vi "Lift Init.vi"   [LabVIEW 2014]
uses:
  Begin/Global Variables.vi
  Begin/Global RefNums.vi
types:
  T1 = typedef "WPI_SwitchDevRef.ctl" = cluster{"DevStatus":errorcluster, "DIO Channel":T2, "Controller":T3, "CntIndex":T4, "Normally Closed":bool}
  T2 = typedef "FPGA_DIOChannel.ctl" = enum8{"DIO 0", "DIO 1", "DIO 2", "DIO 3", "DIO 4", "DIO 5", "DIO 6", "DIO 7", "DIO 8", "DIO 9", "DIO MXP 0", "DIO MXP 1", "DIO MXP 2", "DIO MXP 3", "DIO MXP 4", "DIO MXP 5", "DIO MXP 6", "DIO MXP 7", "DIO MXP 8", "DIO MXP 9", "DIO MXP 10", "DIO MXP 11", "DIO MXP 12", "DIO MXP 13", "DIO MXP 14", "DIO MXP 15", "Invalid"}
  T3 = typedef "FPGA_TypedefDigitalModule.ctl" = enum16{"Controller 1"}
  T4 = typedef "FPGA_CounterCtrSystemIndex.ctl" = enum8{"Ctr 0", "Ctr 1", "Ctr 2", "Ctr 3", "Ctr 4", "Ctr 5", "Ctr 6", "Ctr 7", "Invalid"}
  T5 = typedef "WPI_MotorControlDeviceRef.ctl" = cluster{"DeviceStatus":errorcluster, "Type":T6, "PWM":cluster{"Controller":T3, "PWM Channel":T7, "DeadBand":T8}, "CAN":cluster{"Device Number":u8, "Control Mode":T9, "Semaphore":T10, "Max Vout":dbl, "TalonSRX Control Mode":T11}, "Invert":bool, "TransformRef":T12, "InvTransformRef":T12}
  T6 = typedef "WPI_MotorControlType.ctl" = enum16{"PWM", "CAN", "CANTalonSRX"}
  T7 = typedef "FPGA_DIOPWMChannel.ctl" = enum8{"PWM 0", "PWM 1", "PWM 2", "PWM 3", "PWM 4", "PWM 5", "PWM 6", "PWM 7", "PWM 8", "PWM 9", "PWM MXP 0", "PWM MXP 1", "PWM MXP 2", "PWM MXP 3", "PWM MXP 4", "PWM MXP 5", "PWM MXP 6", "PWM MXP 7", "PWM MXP 8", "PWM MXP 9", "Invalid"}
  T8 = typedef "WPI_PWMDeadband.ctl" = cluster{"Name":string, "maxPositivePwm":i32, "minPositivePwm":i32, "centerPwm":i32, "maxNegativePwm":i32, "minNegativePwm":i32, "angularRange":u16}
  T9 = typedef "WPI_CANJaguar_ControlMode.ctl" = enum8{"Percent VBus", "Current", "Speed", "Position", "Voltage"}
  T10 = typedef "Semaphore RefNum" = refnum<k1>
  T11 = typedef "WPI_CANTalonSRX_APIControlMode.ctl" = enum8{"Percent VBus", "Speed", "Position", "Slave", "Unchanged / Invalid"}
  T12 = typedef "WPI_PWMTransform_ConPane.ctl" = refnum<vi>
  T13 = typedef "WPI_EncoderDevRef.ctl" = cluster{"DevStatus":errorcluster, "EncoderIndex":T14, "CounterIndex":T4, "DistancePerCount":dbl, "Decoding Type":T15}
  T14 = typedef "FPGA_EncoderIdx.ctl" = enum8{"Enc 0", "Enc 1", "Enc 2", "Enc 3", "Enc 4", "Enc 5", "Enc 6", "Enc 7", "Invalid"}
  T15 = typedef "WPI_EncoderType.ctl" = enum16{"1x", "2x", "4x"}
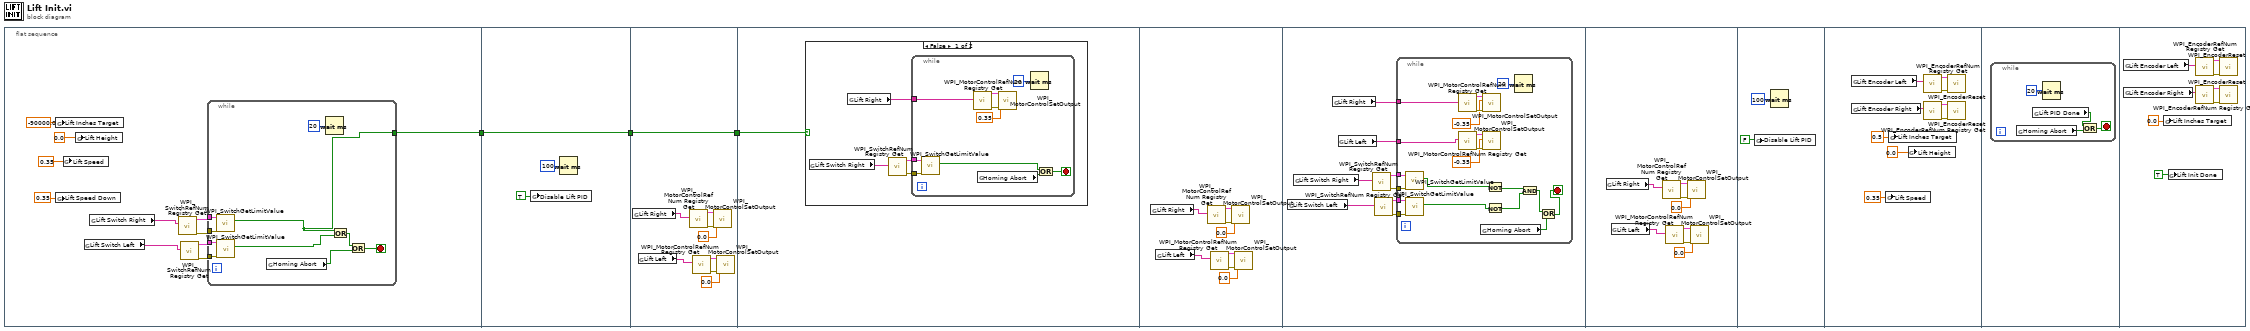
[diagram p0: block diagram]
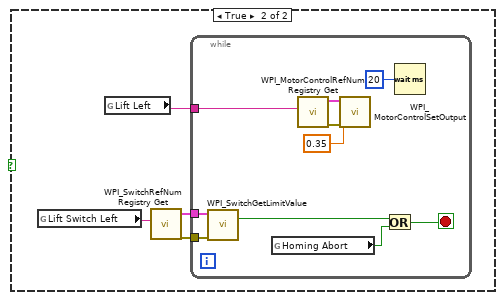
[diagram p2: hidden frame]
diagram:
  n1 = flat-sequence {
    tunnel: [w5] -> w2
    tunnel: w2 -> [w27]
    tunnel: [w27] -> w1
    tunnel: w1 -> [w36]
    tunnel: [w36] -> w3
    tunnel: w3 -> [w37]
    frame #0 {
      n2 = global write "Global Variables.vi" "Lift Inches Target"(-90000.0 ("Lift Inches Target")) -> ()
      n3 = global write "Global Variables.vi" "Lift Speed Down"(0.35 ("Lift Speed Down")) -> ()
      n4 = global write "Global Variables.vi" "Lift Speed"(0.35 ("t")) -> ()
      n5 = global write "Global Variables.vi" "Lift Height"(0.0 ("Lift Inches Target")) -> ()
      n6 = global read "Global RefNums.vi" "Lift Switch Left"() -> (w10:string)
      n7 = global read "Global RefNums.vi" "Lift Switch Right"() -> (w11:string)
      n8 = call <vilib>:"WPI_SwitchRefNum Registry Get.vi"("refnum name"=w11) -> ("error out"=w8:errorcluster, "SwitchDevRef"=w9:T1)  [unwired: 9 in]
      n9 = call <vilib>:"WPI_SwitchRefNum Registry Get.vi"("refnum name"=w10) -> ("error out"=w7:errorcluster, "SwitchDevRef"=w6:T1)  [unwired: 9 in]
      n10 = while {
        tunnel: w9 -> [w23]
        tunnel: w8 -> [w22]
        tunnel: w6 -> [w21]
        tunnel: w7 -> [w20]
        tunnel: [w18] -> w5
        stop <- w15 stop-if-true
        n11 = call <vilib>:"WPI_SwitchGetLimitValue.vi"("error in (no error)"=w22, "SwitchDevRef"=w23) -> ("Switch Pressed"=w18:bool)  [unwired: 7 in, 2 out]
        n12 = call <vilib>:"WPI_SwitchGetLimitValue.vi"("error in (no error)"=w20, "SwitchDevRef"=w21) -> ("Switch Pressed"=w19:bool)  [unwired: 7 in, 2 out]
        n13 = global read "Global Variables.vi" "Homing Abort"() -> (w17:bool)
        n14 = Wait (ms)(milliseconds to wait=u32 20) -> ()  [unwired: 1 out]
        n15 = Or(x=w18, y=w19) -> (x .or. y?=w16:bool)
        n16 = Or(x=w16, y=w17) -> (x .or. y?=w15:bool)
      }
    }
    frame #1 {
      n17 = global write "Global Variables.vi" "Disable Lift PID"(TRUE ("Disable Lift PID")) -> ()
      n18 = Wait (ms)(milliseconds to wait=u32 100) -> ()  [unwired: 1 out]
    }
    frame #2 {
      n19 = global read "Global RefNums.vi" "Lift Right"() -> (w33:string)
      n20 = global read "Global RefNums.vi" "Lift Left"() -> (w29:string)
      n21 = call <vilib>:"WPI_MotorControlRefNum Registry Get.vi"("refnum name"=w33) -> ("error out"=w35:errorcluster, "MotorControlDevRef"=w32:T5)  [unwired: 9 in]
      n22 = call <vilib>:"WPI_MotorControlRefNum Registry Get.vi"("refnum name"=w29) -> ("error out"=w31:errorcluster, "MotorControlDevRef"=w28:T5)  [unwired: 9 in]
      n23 = call <vilib>:"WPI_MotorControlSetOutput.vi"("error in (no error)"=w35, "Output"=0.0, "MotorControlDevRef"=w32) -> ()  [unwired: 6 in, 3 out]
      n24 = call <vilib>:"WPI_MotorControlSetOutput.vi"("error in (no error)"=w31, "Output"=0.0, "MotorControlDevRef"=w28) -> ()  [unwired: 6 in, 3 out]
    }
    frame #3 {
      n25 = case shown="False" w37 {
        frame False {
          n26 = global read "Global RefNums.vi" "Lift Switch Right"() -> (w40:string)
          n27 = global read "Global RefNums.vi" "Lift Right"() -> (w41:string)
          n28 = call <vilib>:"WPI_SwitchRefNum Registry Get.vi"("refnum name"=w40) -> ("error out"=w38:errorcluster, "SwitchDevRef"=w39:T1)  [unwired: 9 in]
          n29 = while {
            tunnel: w41 -> [w48]
            tunnel: w39 -> [w47]
            tunnel: w38 -> [w46]
            stop <- w42 stop-if-true
            n30 = call <vilib>:"WPI_SwitchGetLimitValue.vi"("error in (no error)"=w46, "SwitchDevRef"=w47) -> ("Switch Pressed"=w43:bool)  [unwired: 7 in, 2 out]
            n31 = call <vilib>:"WPI_MotorControlRefNum Registry Get.vi"("refnum name"=w48) -> ("error out"=w50:errorcluster, "MotorControlDevRef"=w51:T5)  [unwired: 9 in]
            n32 = global read "Global Variables.vi" "Homing Abort"() -> (w44:bool)
            n33 = call <vilib>:"WPI_MotorControlSetOutput.vi"("error in (no error)"=w50, "Output"=0.35, "MotorControlDevRef"=w51) -> ()  [unwired: 6 in, 3 out]
            n34 = Wait (ms)(milliseconds to wait=u32 20) -> ()  [unwired: 1 out]
            n35 = Or(x=w43, y=w44) -> (x .or. y?=w42:bool)
          }
        }
        frame True {
          n36 = global read "Global RefNums.vi" "Lift Switch Left"() -> (w53:string)
          n37 = global read "Global RefNums.vi" "Lift Left"() -> (w52:string)
          n38 = call <vilib>:"WPI_SwitchRefNum Registry Get.vi"("refnum name"=w53) -> ("error out"=w54:errorcluster, "SwitchDevRef"=w55:T1)  [unwired: 9 in]
          n39 = while {
            tunnel: w55 -> [w62]
            tunnel: w54 -> [w61]
            tunnel: w52 -> [w60]
            stop <- w58 stop-if-true
            n40 = call <vilib>:"WPI_SwitchGetLimitValue.vi"("error in (no error)"=w61, "SwitchDevRef"=w62) -> ("Switch Pressed"=w57:bool)  [unwired: 7 in, 2 out]
            n41 = global read "Global Variables.vi" "Homing Abort"() -> (w56:bool)
            n42 = call <vilib>:"WPI_MotorControlRefNum Registry Get.vi"("refnum name"=w60) -> ("error out"=w64:errorcluster, "MotorControlDevRef"=w65:T5)  [unwired: 9 in]
            n43 = call <vilib>:"WPI_MotorControlSetOutput.vi"("error in (no error)"=w64, "Output"=0.35, "MotorControlDevRef"=w65) -> ()  [unwired: 6 in, 3 out]
            n44 = Or(x=w57, y=w56) -> (x .or. y?=w58:bool)
            n45 = Wait (ms)(milliseconds to wait=u32 20) -> ()  [unwired: 1 out]
          }
        }
      }
    }
    frame #4 {
      n46 = global read "Global RefNums.vi" "Lift Right"() -> (w71:string)
      n47 = global read "Global RefNums.vi" "Lift Left"() -> (w67:string)
      n48 = call <vilib>:"WPI_MotorControlRefNum Registry Get.vi"("refnum name"=w71) -> ("error out"=w73:errorcluster, "MotorControlDevRef"=w70:T5)  [unwired: 9 in]
      n49 = call <vilib>:"WPI_MotorControlRefNum Registry Get.vi"("refnum name"=w67) -> ("error out"=w69:errorcluster, "MotorControlDevRef"=w66:T5)  [unwired: 9 in]
      n50 = call <vilib>:"WPI_MotorControlSetOutput.vi"("error in (no error)"=w73, "Output"=0.0, "MotorControlDevRef"=w70) -> ()  [unwired: 6 in, 3 out]
      n51 = call <vilib>:"WPI_MotorControlSetOutput.vi"("error in (no error)"=w69, "Output"=0.0, "MotorControlDevRef"=w66) -> ()  [unwired: 6 in, 3 out]
    }
    frame #5 {
      n52 = global read "Global RefNums.vi" "Lift Switch Left"() -> (w74:string)
      n53 = global read "Global RefNums.vi" "Lift Switch Right"() -> (w80:string)
      n54 = global read "Global RefNums.vi" "Lift Right"() -> (w81:string)
      n55 = global read "Global RefNums.vi" "Lift Left"() -> (w77:string)
      n56 = call <vilib>:"WPI_SwitchRefNum Registry Get.vi"("refnum name"=w80) -> ("error out"=w78:errorcluster, "SwitchDevRef"=w79:T1)  [unwired: 9 in]
      n57 = call <vilib>:"WPI_SwitchRefNum Registry Get.vi"("refnum name"=w74) -> ("error out"=w75:errorcluster, "SwitchDevRef"=w76:T1)  [unwired: 9 in]
      n58 = while {
        tunnel: w81 -> [w98]
        tunnel: w79 -> [w97]
        tunnel: w78 -> [w96]
        tunnel: w77 -> [w92]
        tunnel: w76 -> [w91]
        tunnel: w75 -> [w90]
        stop <- w82 stop-if-true
        n59 = call <vilib>:"WPI_SwitchGetLimitValue.vi"("error in (no error)"=w96, "SwitchDevRef"=w97) -> ("Switch Pressed"=w87:bool)  [unwired: 7 in, 2 out]
        n60 = call <vilib>:"WPI_SwitchGetLimitValue.vi"("error in (no error)"=w90, "SwitchDevRef"=w91) -> ("Switch Pressed"=w85:bool)  [unwired: 7 in, 2 out]
        n61 = call <vilib>:"WPI_MotorControlRefNum Registry Get.vi"("refnum name"=w98) -> ("error out"=w100:errorcluster, "MotorControlDevRef"=w101:T5)  [unwired: 9 in]
        n62 = call <vilib>:"WPI_MotorControlRefNum Registry Get.vi"("refnum name"=w92) -> ("error out"=w94:errorcluster, "MotorControlDevRef"=w89:T5)  [unwired: 9 in]
        n63 = global read "Global Variables.vi" "Homing Abort"() -> (w84:bool)
        n64 = call <vilib>:"WPI_MotorControlSetOutput.vi"("error in (no error)"=w100, "Output"=-0.35 ("right side  2"), "MotorControlDevRef"=w101) -> ()  [unwired: 6 in, 3 out]
        n65 = call <vilib>:"WPI_MotorControlSetOutput.vi"("error in (no error)"=w94, "Output"=-0.35 ("right side  2"), "MotorControlDevRef"=w89) -> ()  [unwired: 6 in, 3 out]
        n66 = Not(x=w87) -> (.not. x?=w88:bool)
        n67 = Not(x=w85) -> (.not. x?=w86:bool)
        n68 = Wait (ms)(milliseconds to wait=u32 20) -> ()  [unwired: 1 out]
        n69 = And(x=w88, y=w86) -> (x .and. y?=w83:bool)
        n70 = Or(x=w83, y=w84) -> (x .or. y?=w82:bool)
      }
    }
    frame #6 {
      n71 = global read "Global RefNums.vi" "Lift Right"() -> (w107:string)
      n72 = global read "Global RefNums.vi" "Lift Left"() -> (w103:string)
      n73 = call <vilib>:"WPI_MotorControlRefNum Registry Get.vi"("refnum name"=w107) -> ("error out"=w109:errorcluster, "MotorControlDevRef"=w106:T5)  [unwired: 9 in]
      n74 = call <vilib>:"WPI_MotorControlRefNum Registry Get.vi"("refnum name"=w103) -> ("error out"=w105:errorcluster, "MotorControlDevRef"=w102:T5)  [unwired: 9 in]
      n75 = call <vilib>:"WPI_MotorControlSetOutput.vi"("error in (no error)"=w109, "Output"=0.0, "MotorControlDevRef"=w106) -> ()  [unwired: 6 in, 3 out]
      n76 = call <vilib>:"WPI_MotorControlSetOutput.vi"("error in (no error)"=w105, "Output"=0.0, "MotorControlDevRef"=w102) -> ()  [unwired: 6 in, 3 out]
    }
    frame #7 {
      n77 = global write "Global Variables.vi" "Disable Lift PID"(FALSE ("Disable Lift PID")) -> ()
      n78 = Wait (ms)(milliseconds to wait=u32 100) -> ()  [unwired: 1 out]
    }
    frame #8 {
      n79 = global read "Global RefNums.vi" "Lift Encoder Left"() -> (w117:string)
      n80 = global read "Global RefNums.vi" "Lift Encoder Right"() -> (w116:string)
      n81 = global write "Global Variables.vi" "Lift Speed"(0.35 ("Lift Speed")) -> ()
      n82 = global write "Global Variables.vi" "Lift Inches Target"(0.5 ("Lift Inches Target")) -> ()
      n83 = global write "Global Variables.vi" "Lift Height"(0.0 ("Lift Inches Target")) -> ()
      n84 = call <vilib>:"WPI_EncoderRefNum Registry Get.vi"("refnum name"=w117) -> ("error out"=w120:errorcluster, "EncoderDevRef"=w115:T13)  [unwired: 9 in]
      n85 = call <vilib>:"WPI_EncoderRefNum Registry Get.vi"("refnum name"=w116) -> ("error out"=w118:errorcluster, "EncoderDevRef"=w119:T13)  [unwired: 9 in]
      n86 = call <vilib>:"WPI_EncoderReset.vi"("error in (no error)"=w120, "EncoderDevRef"=w115) -> ()  [unwired: 8 in, 2 out]
      n87 = call <vilib>:"WPI_EncoderReset.vi"("error in (no error)"=w118, "EncoderDevRef"=w119) -> ()  [unwired: 8 in, 2 out]
    }
    frame #9 {
      n88 = while {
        stop <- w122 stop-if-true
        n89 = global read "Global Variables.vi" "Homing Abort"() -> (w121:bool)
        n90 = global read "Global Variables.vi" "Lift PID Done"() -> (w123:bool)
        n91 = Wait (ms)(milliseconds to wait=u32 20) -> ()  [unwired: 1 out]
        n92 = Or(x=w123, y=w121) -> (x .or. y?=w122:bool)
      }
    }
    frame #10 {
      n93 = global read "Global RefNums.vi" "Lift Encoder Left"() -> (w131:string)
      n94 = global read "Global RefNums.vi" "Lift Encoder Right"() -> (w132:string)
      n95 = global write "Global Variables.vi" "Lift Inches Target"(0.0 ("Lift Inches Target")) -> ()
      n96 = global write "Global Variables.vi" "Lift Init Done"(TRUE ("Lift Init Done")) -> ()
      n97 = call <vilib>:"WPI_EncoderRefNum Registry Get.vi"("refnum name"=w131) -> ("error out"=w128:errorcluster, "EncoderDevRef"=w127:T13)  [unwired: 9 in]
      n98 = call <vilib>:"WPI_EncoderRefNum Registry Get.vi"("refnum name"=w132) -> ("error out"=w130:errorcluster, "EncoderDevRef"=w129:T13)  [unwired: 9 in]
      n99 = call <vilib>:"WPI_EncoderReset.vi"("error in (no error)"=w128, "EncoderDevRef"=w127) -> ()  [unwired: 8 in, 2 out]
      n100 = call <vilib>:"WPI_EncoderReset.vi"("error in (no error)"=w130, "EncoderDevRef"=w129) -> ()  [unwired: 8 in, 2 out]
    }
  }
